vi "UDP Data Link - Configuration Utilities - Set Rx Channels.vi"(8 "error in (no error)":errorcluster, 9 "Rx Channel Paths":string[](array[string]), 10 "Rx Channel Names":string[](array[string]), 11 "Item Ref in":T1 format="%.0x") -> (0 "error out":errorcluster, 3 "Item Ref out":T1=18446744073709551615 format="%.0x")   [LabVIEW 2012, in "UDP Data Link System Explorer.lvlib"]
uses:
  UDP Data Link System Explorer.lvlib
  <vilib>/NI Veristand/Custom Device API/Custom Device Item Ref.ctl
  Shared/UDP Data Link Global.vi
  <vilib>/NI Veristand/Custom Device API/Get Item Property (Dependent Node Pointer).vi
  <vilib>/NI Veristand/Custom Device Tools/Custom Device Utility Library/Custom Device Utility Library.lvlib
  <vilib>/NI Veristand/Custom Device API/Custom Device API.lvlib
  Shared/UDP Data Link Shared.lvlib
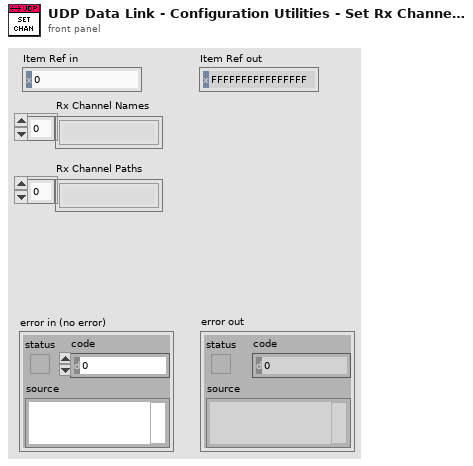
[diagram p1: front panel]
types:
  T1 = typedef "Custom Device API.lvlib/Custom Device Item Ref.ctl" = u64
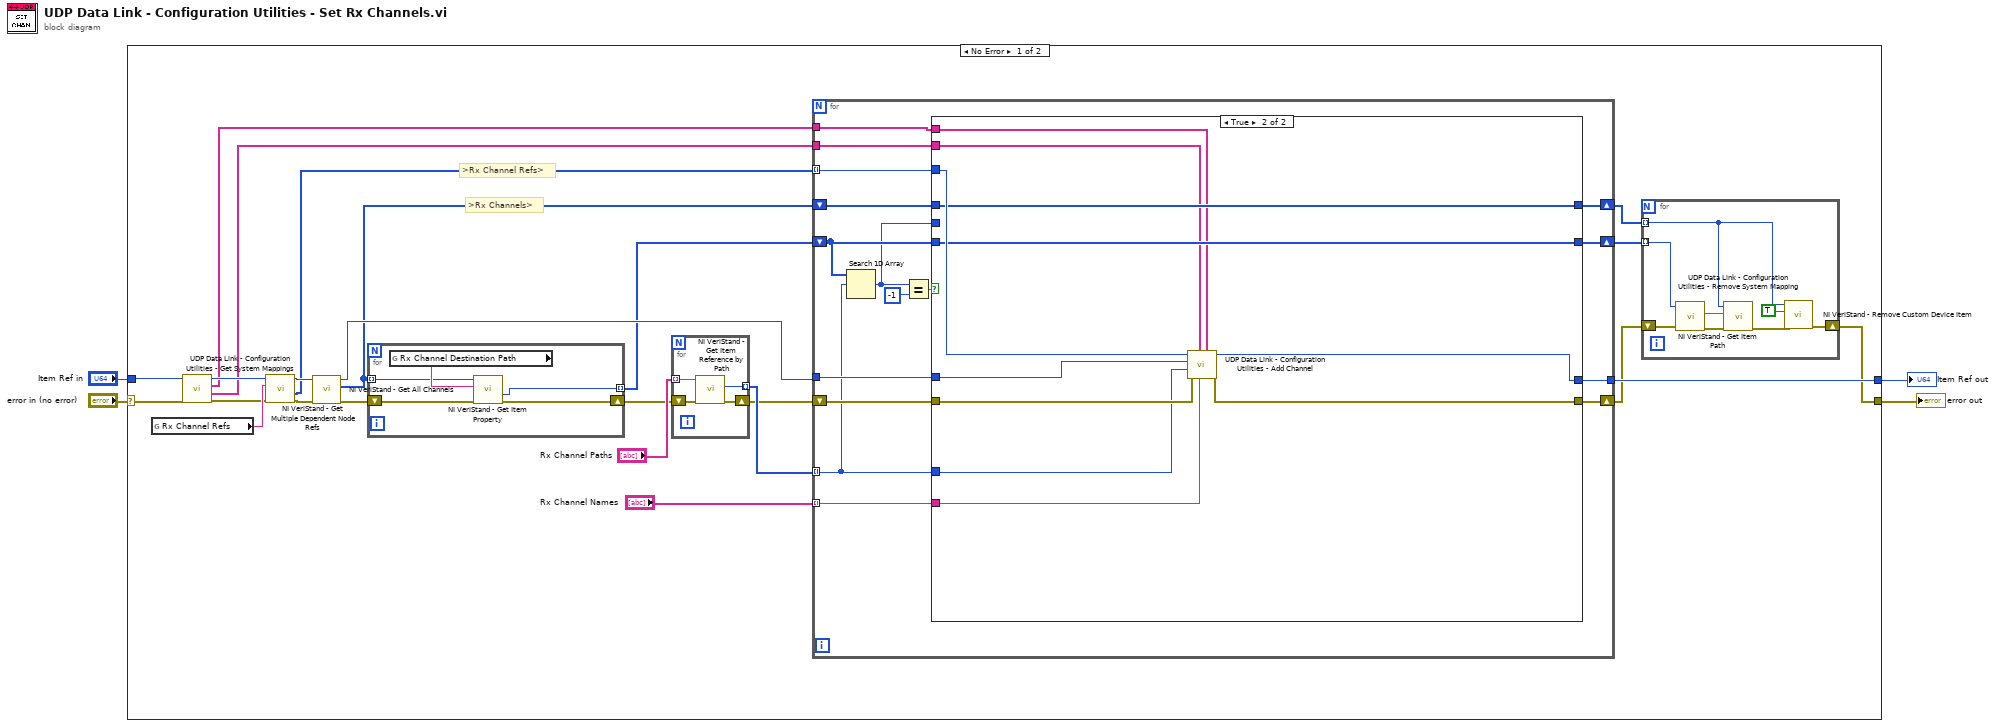
[diagram p0: block diagram]
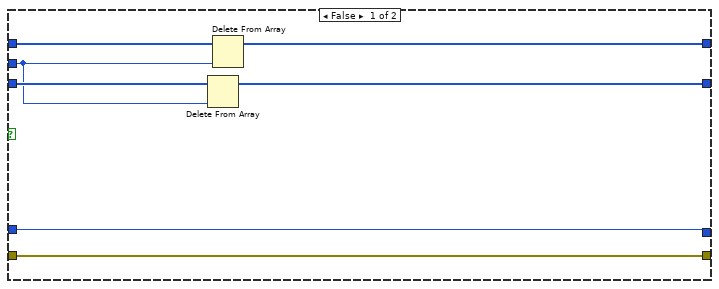
[diagram p2: hidden frame]
diagram:
  n1 = case shown="No Error" "error in (no error)" {
    selector: "error in (no error)" -> [w10 w80]
    tunnel: "Item Ref in" -> [w7 w81]
    tunnel: [w25 w81] -> w2
    tunnel: [w18 w80] -> w1
    frame No Error {
      # ">Rx Channels>"
      # ">Rx Channel Refs>"
      n2 = global read "UDP Data Link Global.vi" "Rx Channel Refs"() -> (w23:string)
      n3 = call "UDP Data Link - Configuration Utilities - Get System Mappings.vi"("error in (no error)"=w10, "Item Ref in"=w7) -> ("error out"=w9:errorcluster, "Channel Path Destinations"=w5:string[], "Channel Path Sources"=w6:string[], "Item Ref out"=w8:T1)  [unwired: 6 in]
      n4 = call <vilib>:"NI VeriStand - Get Multiple Dependent Node Refs.vi"("error in (no error)"=w9, "Base Property Name"=w23, "Item Ref in"=w8) -> ("error out"=w24:errorcluster, "Dependent Node Refs"=w21:T1[], "Item Ref out"=w22:T1)  [unwired: 6 in]
      n5 = call <vilib>:"NI VeriStand - Get All Channels.vi"("error in"=w24, "Section Ref in"=w22) -> ("error out"=w28:errorcluster, "Channel Refs"=w20:T1[], "Section Ref out"=w26:T1)  [unwired: 6 in, 1 out]
      n6 = for {
        tunnel: w20 -> [w78] mode=indexing
        tunnel: [w76] -> w16 mode=indexing
        shift-right: [w75] -> w13
        shift-left: w28 -> [w77]
        n7 = global read "UDP Data Link Global.vi" "Rx Channel Destination Path"() -> (w79:string)
        n8 = call-poly <vilib>:"NI VeriStand - Get Item Property.vi"("error in (no error)"=w77, "Property Name"=w79, "Item Ref in"=w78) -> ("error out"=w75:errorcluster, "Dependent Node Ref"=w76:T1)  [unwired: 5 in, 2 out]
      }
      n9 = for {
        tunnel: "Rx Channel Paths" -> [w32] mode=indexing
        tunnel: [w31] -> w14 mode=indexing
        shift-right: [w29] -> w12
        shift-left: w13 -> [w30]
        n10 = call <vilib>:"NI VeriStand - Get Item Reference by Path.vi"("error in (no error)"=w30, "Item Path in"=w32) -> ("error out"=w29:errorcluster, "Item Ref"=w31:T1)  [unwired: 6 in, 2 out]
      }
      n11 = for {
        tunnel: w14 -> [w51] mode=indexing
        shift-right: [w50] -> w19
        shift-left: w12 -> [w54]
        tunnel: w26 -> [w53]
        tunnel: "Rx Channel Names" -> [w52] mode=indexing
        tunnel: w21 -> [w49] mode=indexing
        tunnel: [w48] -> w25
        shift-right: [w46] -> w17
        shift-left: w20 -> [w47]
        shift-right: [w44] -> w11
        shift-left: w16 -> [w45]
        tunnel: w6 -> [w41]
        tunnel: w5 -> [w42]
        n12 = Search 1D Array(1D array=w45, element=w51) -> (index of element=w43:i32)  [unwired: 1 in]
        n13 = Equal?(x=w43, y=-1) -> (x = y?=w55:bool)
        n14 = case shown="True" w55 {
          tunnel: w54 -> [w57 w74]
          tunnel: w53 -> [w58 w73]
          tunnel: w52 -> [_ w66]
          tunnel: w51 -> [_ w67]
          tunnel: [w57 w68] -> w50
          tunnel: w49 -> [_ w72]
          tunnel: [w58 w71] -> w48
          tunnel: w47 -> [w63 w70]
          tunnel: [w62 w70] -> w46
          tunnel: w43 -> [w59 _]
          tunnel: w45 -> [w61 w69]
          tunnel: [w60 w69] -> w44
          tunnel: w42 -> [_ w65]
          tunnel: w41 -> [_ w64]
          frame False {
            n15 = Delete From Array(array=w61, index=w59) -> (array with subset deleted=w60:T1[])  [unwired: 1 in, 1 out]
            n16 = Delete From Array(array=w63, index=w59) -> (array with subset deleted=w62:T1[])  [unwired: 1 in, 1 out]
          }
          frame True {
            n17 = call "UDP Data Link - Configuration Utilities - Add Channel.vi"("Channel Path Sources"=w64, "Rx Channel Name"=w66, "Channel Path Destinations"=w65, "error in (no error)"=w74, "Rx Channel Ref"=w67, "Rx Section Ref in"=w73, "Dependent Node Ref"=w72) -> ("error out"=w68:errorcluster, "Rx Section Ref in"=w71:T1)  [unwired: 3 in]
          }
        }
      }
      n18 = for {
        shift-right: [w40] -> w18
        shift-left: w19 -> [w38]
        tunnel: w17 -> [w33] mode=indexing
        tunnel: w11 -> [w34] mode=indexing
        n19 = call <vilib>:"NI VeriStand - Get Item Path.vi"("error in (no error)"=w38, "Item Ref in"=w34) -> ("error out"=w37:errorcluster, "Path"=w35:string)  [unwired: 6 in, 2 out]
        n20 = call "UDP Data Link - Configuration Utilities - Remove System Mapping.vi"("error in (no error)"=w37, "Channel Path Destination"=w35, "Item Ref in"=w33) -> ("error out"=w36:errorcluster)  [unwired: 7 in, 1 out]
        n21 = call <vilib>:"NI VeriStand - Remove Custom Device Item.vi"("error in (no error)"=w36, "Force Delete (F)"=TRUE, "Item Ref in"=w33) -> ("error out"=w40:errorcluster)  [unwired: 7 in, 1 out]
      }
    }
    frame Error {
    }
  }
  "Item Ref out" <- w2
  "error out" <- w1
